vi "실습5.vi"() -> ()   [LabVIEW 2014]
panel:
  out "웨이브폼 차트":dbl
  in  "대기 시간(ms)":u32
  in  "vi 경로":path
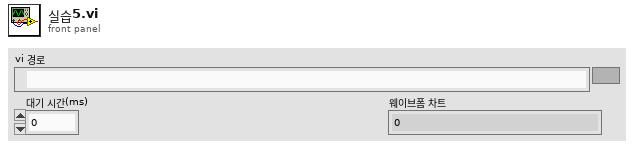
[diagram p1: front panel]
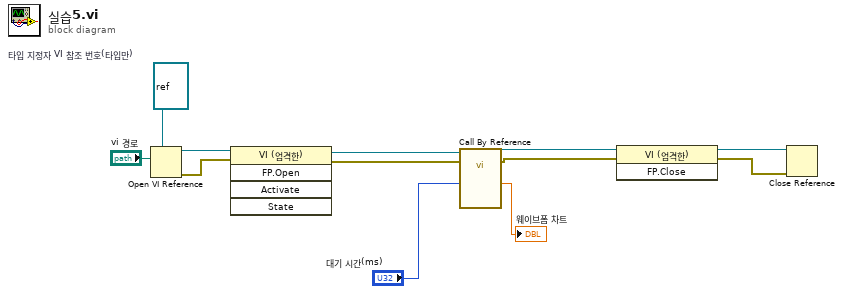
[diagram p0: block diagram]
diagram:
  w11 = refnum<vi> refnum  # 타입 지정자 VI 참조 번호(타입만)
  n1 = Open VI Reference(type specifier VI Refnum (for type only)=w11, vi path="vi 경로") -> (vi reference=w8:refnum<vi>, error out=w7:errorcluster)  [unwired: 4 in]
  n2 = invoke class="VI (엄격한)" method="FP.Open"(reference=w8, error in=w7) -> (reference out=w6:refnum<vi>, error out=w5:errorcluster)  [unwired: 3 in, 3 out]
  n3 = call-by-ref "?"(reference=w6, error in=w5, "대기 시간(ms)"="대기 시간(ms)") -> (reference out=w4:refnum<vi>, error out=w3:errorcluster, "웨이브폼 차트"=→"웨이브폼 차트":dbl)  [unwired: 10 in]
  n4 = invoke class="VI (엄격한)" method="FP.Close"(reference=w4, error in=w3) -> (reference out=w2:refnum<vi>, error out=w1:errorcluster)  [unwired: 1 in, 1 out]
  n5 = Close Reference(reference=w2, error in (no error)=w1) -> ()  [unwired: 1 out]
